vi "lv-ros-bridge_WRITE.vi"(10 "rosbridge port":u16=9090, 11 "rosbridge server IP":string="192.168.164.128") -> (0 "error out":errorcluster)   [LabVIEW 2015]
uses:
  Control  rossss.ctl
  <vilib>/Utility/inputDevices.llb/joystickAcquire.vi
  <vilib>/Utility/inputDevices.llb/closeJoystick.vi
  <vilib>/Intelligent Energy/WebSockets API/WebSockets/WebSockets.lvlib
panel:
  in  "msg.layout.dim":T1(array[cluster])
  out "output cluster":T2={"op"="publish", "topic"="", "msg"={"layout"={"dim"=[]}, "data"=[]}}
  out "Opcode 2":u8
  out "Data 2":string
  out "concatenated string":string
  in  "type":string="std_msgs/Int32MultiArray"
  out "direction info":T3
  out "button info":T4
  out "axis info":T5
  in  "device index":i32
  in  "Topic to write":string="rio"
  in  "format wiadomości":T2={"op"="publish", "topic"="", "msg"={"layout"={"dim"=[]}, "data"=[]}}
  out "raw JSON frame":string
  in  "stop":bool
  # "ZAWSZE UŻYWAJ STOPU!!!"
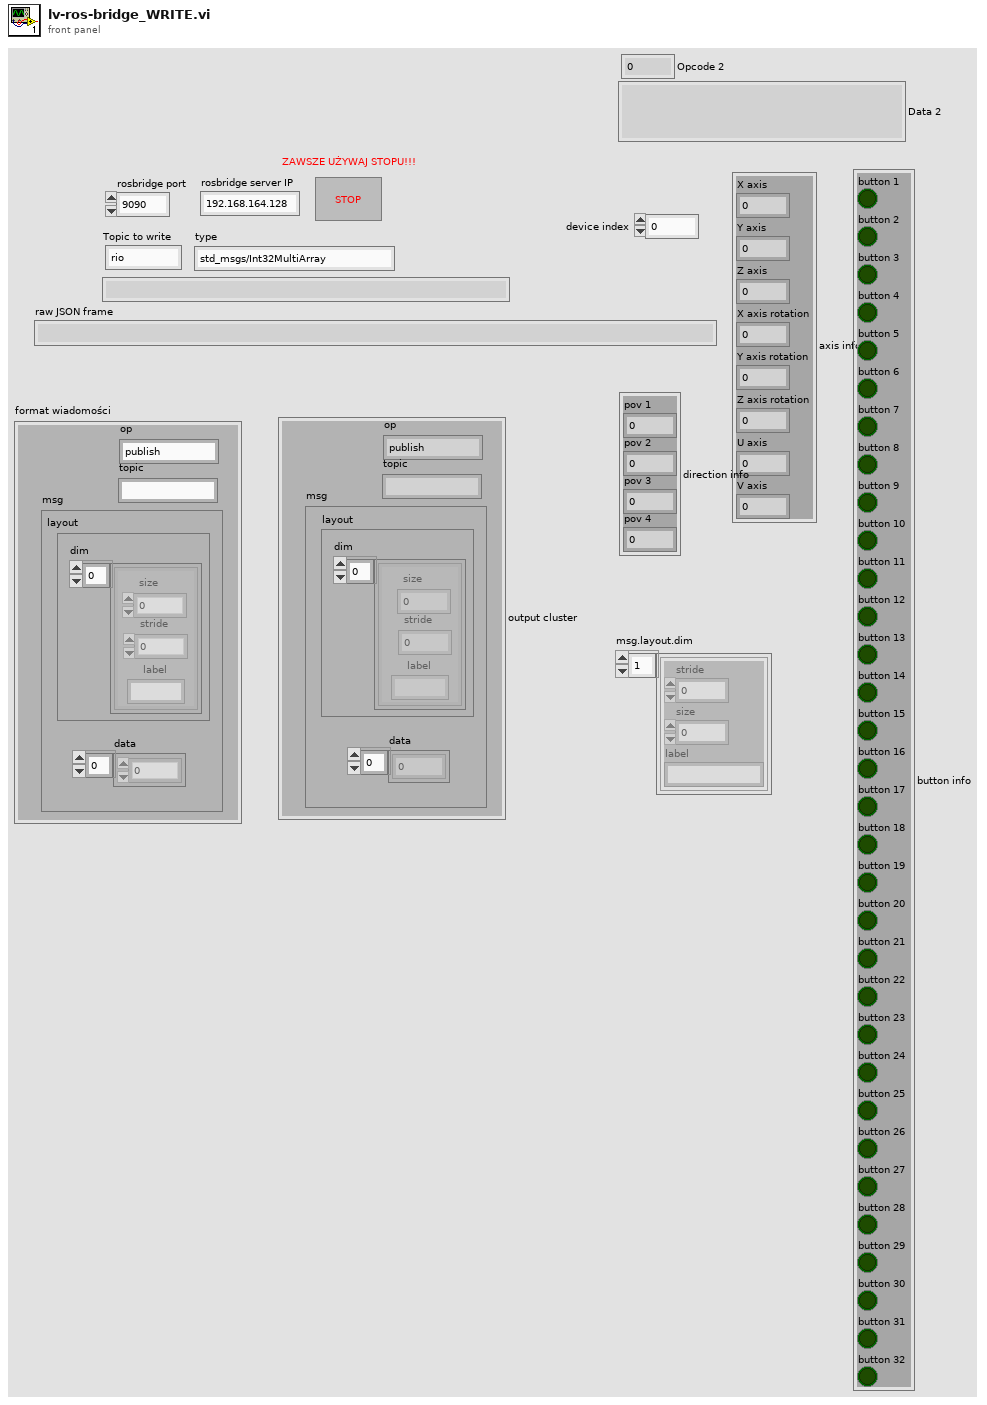
[diagram p1: front panel]
types:
  T1 = cluster{"stride":i16, "size":i16, "label":string}[]
  T2 = typedef "Control  rossss.ctl" = cluster{"op":string, "topic":string, "msg":cluster{"layout":cluster{"dim":cluster{"stride":i16, "size":i16, "label":string}[]}, "data":i32[]}}
  T3 = cluster{"pov 1":i32, "pov 2":i32, "pov 3":i32, "pov 4":i32}
  T4 = cluster{"button 1":bool, "button 2":bool, "button 3":bool, "button 4":bool, "button 5":bool, "button 6":bool, "button 7":bool, "button 8":bool, "button 9":bool, "button 10":bool, "button 11":bool, "button 12":bool, "button 13":bool, "button 14":bool, "button 15":bool, "button 16":bool, "button 17":bool, "button 18":bool, "button 19":bool, "button 20":bool, "button 21":bool, "button 22":bool, "button 23":bool, "button 24":bool, "button 25":bool, "button 26":bool, "button 27":bool, "button 28":bool, "button 29":bool, "button 30":bool, "button 31":bool, "button 32":bool}
  T5 = cluster{"X axis":i32, "Y axis":i32, "Z axis":i32, "X axis rotation":i32, "Y axis rotation":i32, "Z axis rotation":i32, "U axis":i32, "V axis":i32}
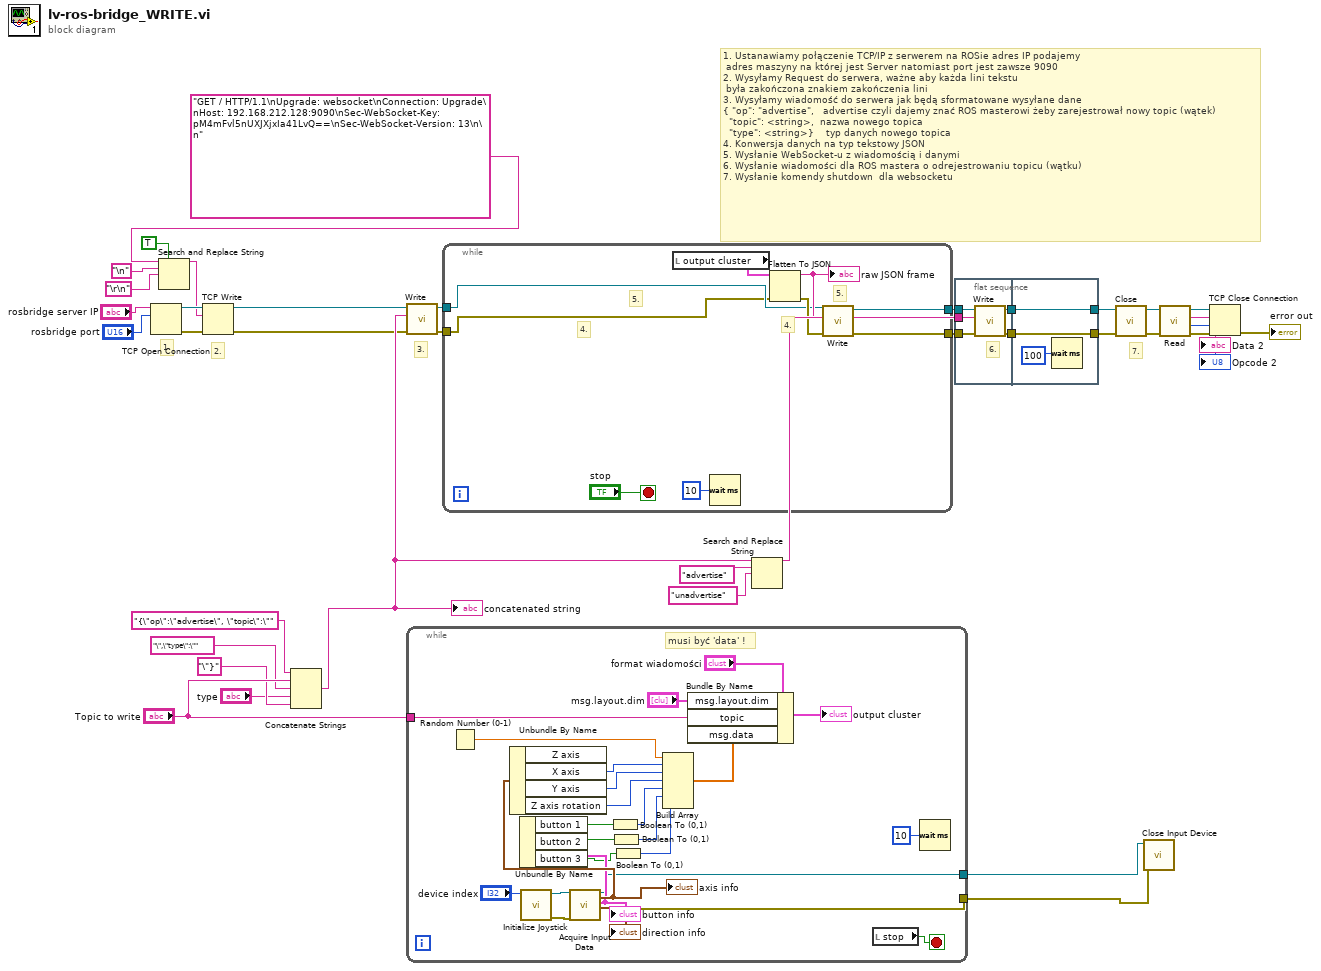
[diagram p0: block diagram]
diagram:
  # "1. Ustanawiamy połączenie TCP/IP z serwerem na ROSie adres IP podajemy\n adres maszyny na której jest Server natomiast port jest zawsze 9090\n2. Wysyłamy Request do serwera, ważne aby każda lini tekstu\n była zakończona znakiem zakończenia lini\n3. Wysyłamy wiadomość do serwera jak będą sformatowane wysyłane dane \n{ \"op\": \"advertise\",   advertise czyli dajemy znać ROS masterowi żeby zarejestrował nowy topic (wątek)\n  \"topic\": <string>,  nazwa nowego topica \n  \"type\": <string>}    typ danych nowego topica\n4. Konwersja danych na typ tekstowy JSON\n5. Wysłanie WebSocket-u z wiadomością i danymi\n6. Wysłanie wiadomości dla ROS mastera o odrejestrowaniu topicu (wątku)\n7. Wysłanie komendy shutdown  dla websocketu"
  # "7."
  # "3."
  # "2."
  # "1."
  n1 = TCP Open Connection(address="rosbridge server IP", remote port or service name="rosbridge port") -> (connection ID=w14:refnum<k5>, error out=w13:errorcluster)  [unwired: 3 in]
  n2 = Search and Replace String(replace all?=TRUE ("replace all? (F)"), input string="GET / HTTP/1.1\nUpgrade: websocket\nConnection: Upgrade\nHost: 192.168.212.128:9090\nSec-WebSocket-Key: pM4mFvl5nUXJXjxIa41LvQ==\nSec-WebSocket-Version: 13\n\n", search string="\n", replace string="\r\n") -> (result string=w12:string)  [unwired: 4 in, 3 out]
  n3 = TCP Write(connection ID=w14, data in=w12, error in (no error)=w13) -> (connection ID out=w2:refnum<k5>, error out=w1:errorcluster)  [unwired: 1 in, 1 out]
  n4 = Concatenate Strings("{\"op\":\"advertise\", \"topic\":\"", "Topic to write", "\",\"type\":\"", "type", "\"}") -> (w32:string)
  "concatenated string" <- w32
  n5 = call <vilib>:"Write.vi"("error in (no error)"=w1, "Data"=w32, "WebSocket Connection in"=w2) -> ("error out"=w26:errorcluster, "WebSocket Connection out"=w25:refnum<k5>)  [unwired: 7 in]
  n6 = while {
    tunnel: "Topic to write" -> [w60]
    tunnel: [w43] -> w31
    tunnel: [w42] -> w30
    stop <- w61 stop-if-true
    # "musi być 'data' !"
    n7 = Random Number (0-1)() -> (number: 0 to 1=w40:dbl)
    n8 = call <vilib>:"Initialize Joystick.vi"("device index"="device index") -> ("error out"=w55:errorcluster, "device ID"=w56:refnum<k1>)  [unwired: 9 in]
    n9 = call-poly <vilib>:"Acquire Input Data.vi"("device ID"=w56, "error in (no error)"=w55) -> ("device ID"=w43:refnum<k1>, "axis info"=w54:T5, "button info"=w50:T4, "direction info"=→"direction info":T3, "error out"=w42:errorcluster)  [unwired: 13 in]
    "axis info" <- w54
    "button info" <- w50
    n10 = Unbundle By Name(w54) -> ("X axis"=w53:i32, "Y axis"=w52:i32, "Z axis rotation"=w51:i32)  [unwired: 1 out]
    n11 = Unbundle By Name(w50) -> ("button 1"=w47:bool, "button 2"=w48:bool, "button 3"=w49:bool)
    n12 = Boolean To (0,1)(Boolean=w47) -> (0, 1=w46:i16)
    n13 = Boolean To (0,1)(Boolean=w48) -> (0, 1=w45:i16)
    n14 = Boolean To (0,1)(Boolean=w49) -> (0, 1=w44:i16)
    n15 = Build Array(w40, w53, w52, w51, w46, w45, w44) -> (w39:dbl[])
    n16 = Bundle By Name(cluster="format wiadomości", "msg.layout.dim"="msg.layout.dim", "topic"=w60, "msg.data"=w39) -> (→"output cluster":T2)
    n17 = local read "stop"() -> (w61:bool)
    n18 = Wait (ms)(milliseconds to wait=u32 10) -> ()  [unwired: 1 out]
  }
  n19 = while {
    tunnel: [w71] -> w23
    tunnel: [w70] -> w21
    tunnel: w25 -> [w64]
    tunnel: w26 -> [w63]
    stop <- "stop" stop-if-true
    # "5."
    # "4."
    # "5."
    # "4."
    n20 = local read "output cluster"() -> (w66:T2)
    n21 = Wait (ms)(milliseconds to wait=u32 10) -> ()  [unwired: 1 out]
    n22 = Flatten To JSON(anything=w66, error in (no error)=w63) -> (JSON string=w67:string, 11:w65:errorcluster)  [unwired: 1 in]
    "raw JSON frame" <- w67
    n23 = call <vilib>:"Write.vi"("error in (no error)"=w65, "Data"=w67, "WebSocket Connection in"=w64) -> ("error out"=w70:errorcluster, "WebSocket Connection out"=w71:refnum<k5>)  [unwired: 7 in]
  }
  n24 = Search and Replace String(input string=w32, search string="advertise", replace string="unadvertise" ("search string")) -> (result string=w11:string)  [unwired: 5 in, 3 out]
  n25 = flat-sequence {
    tunnel: w23 -> [w76]
    tunnel: w21 -> [w75]
    tunnel: w11 -> [w74]
    tunnel: [w73] -> w29
    tunnel: [w72] -> w28
    tunnel: [w78] -> w22
    tunnel: [w79] -> w24
    tunnel: w29 -> [w79]
    tunnel: w28 -> [w78]
    frame #0 {
      # "6."
      n26 = call <vilib>:"Write.vi"("error in (no error)"=w75, "Data"=w74, "WebSocket Connection in"=w76) -> ("error out"=w72:errorcluster, "WebSocket Connection out"=w73:refnum<k5>)  [unwired: 7 in]
    }
    frame #1 {
      n27 = Wait (ms)(milliseconds to wait=u32 100) -> ()  [unwired: 1 out]
    }
  }
  n28 = call <vilib>:"Close.vi"("error in (no error)"=w22, "WebSocket Connection in"=w24) -> ("error out"=w7:errorcluster, "WebSocket Connection in"=w8:refnum<k5>)  [unwired: 8 in]
  n29 = call-poly <vilib>:"Close Input Device.vi"("error in (no error)"=w30, "device ID"=w31) -> ()  [unwired: 8 in, 1 out]
  n30 = call <vilib>:"Read.vi"("error in (no error)"=w7, "WebSocket Connection in"=w8) -> ("error out"=w6:errorcluster, "Opcode"=→"Opcode 2":u8, "Data"=→"Data 2":string, "WebSocket Connection out"=w5:refnum<k5>)  [unwired: 6 in]
  n31 = TCP Close Connection(connection ID=w5, error in (no error)=w6) -> (error out=→"error out":errorcluster)  [unwired: 1 in, 1 out]
